vi "zero.out.and.convert.vi"(11 "Data":T1={"enabled"=[FALSE, FALSE, FALSE, FALSE, FALSE, FALSE, FALSE, FALSE], "byte"=[0, 0, 0, 0, 0, 0, 0, 0]} {"byte" format="%.0x"}) -> (2 "u64.be":u64 format="%.0x", 3 "Num.of.True":u8)   [LabVIEW 2020, in "fpganow.common.fpga.lvlib"]
uses:
  fpganow.common.fpga.lvlib
  u64.data.ctl
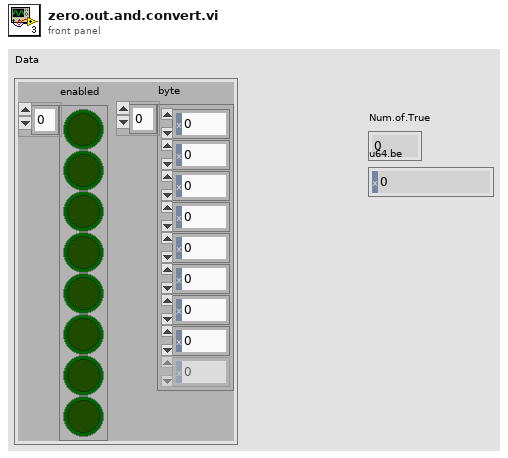
[diagram p1: front panel]
types:
  T1 = typedef "fpganow.common.fpga.lvlib/u64.data.ctl" = cluster{"enabled":bool[], "byte":u8[]}
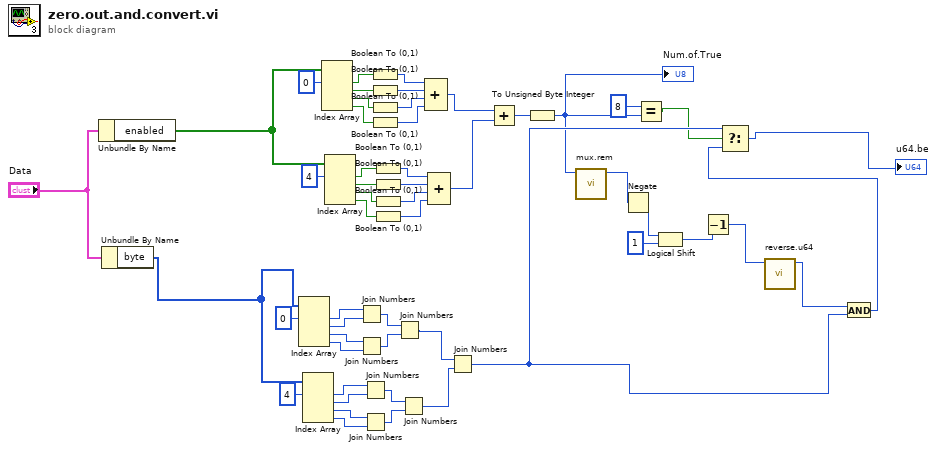
[diagram p0: block diagram]
diagram:
  n1 = Unbundle By Name("Data") -> ("enabled"=w31:bool[])
  n2 = Unbundle By Name("Data") -> ("byte"=w14:u8[])
  n3 = Index Array(array=w14, index #1=0 ("index")) -> (element #1=w29:u8, element #2=w28:u8, element #3=w27:u8, element #4=w26:u8)  [unwired: 3 in]
  n4 = Index Array(array=w14, index #1=4 ("index")) -> (element #1=w21:u8, element #2=w20:u8, element #3=w19:u8, element #4=w18:u8)  [unwired: 3 in]
  n5 = Index Array(array=w31, index #1=0 ("index")) -> (element #1=w33:bool, element #2=w35:bool, element #3=w37:bool, element #4=w40:bool)  [unwired: 3 in]
  n6 = Index Array(array=w31, index #1=4 ("index")) -> (element #1=w43:bool, element #2=w45:bool, element #3=w47:bool, element #4=w50:bool)  [unwired: 3 in]
  n7 = Join Numbers(hi=w29, lo=w28) -> ((hi.lo)=w25:u16)
  n8 = Join Numbers(hi=w27, lo=w26) -> ((hi.lo)=w24:u16)
  n9 = Join Numbers(hi=w21, lo=w20) -> ((hi.lo)=w17:u16)
  n10 = Join Numbers(hi=w19, lo=w18) -> ((hi.lo)=w16:u16)
  n11 = Boolean To (0,1)(Boolean=w33) -> (0, 1=w34:i16)
  n12 = Boolean To (0,1)(Boolean=w35) -> (0, 1=w36:i16)
  n13 = Boolean To (0,1)(Boolean=w37) -> (0, 1=w38:i16)
  n14 = Boolean To (0,1)(Boolean=w40) -> (0, 1=w39:i16)
  n15 = Boolean To (0,1)(Boolean=w43) -> (0, 1=w44:i16)
  n16 = Boolean To (0,1)(Boolean=w45) -> (0, 1=w46:i16)
  n17 = Boolean To (0,1)(Boolean=w47) -> (0, 1=w48:i16)
  n18 = Boolean To (0,1)(Boolean=w50) -> (0, 1=w49:i16)
  n19 = Join Numbers(hi=w25, lo=w24) -> ((hi.lo)=w23:u32)
  n20 = Join Numbers(hi=w17, lo=w16) -> ((hi.lo)=w15:u32)
  n21 = Compound Arithmetic op=ADD(w34, w36, w38, w39) -> (w41:i16)
  n22 = Compound Arithmetic op=ADD(w44, w46, w48, w49) -> (w51:i16)
  n23 = Join Numbers(hi=w23, lo=w15) -> ((hi.lo)=w5:u64)
  n24 = Add(x=w41, y=w51) -> (x+y=w52:i16)
  n25 = To Unsigned Byte Integer(number=w52) -> (unsigned 8bit integer=w4:u8)
  "Num.of.True" <- w4
  n26 = call "mux.rem.vi"("# of existing\nitems 3"=w4) -> ("y"=w11:i8)  [unwired: 10 in]
  n27 = Negate(x=w11) -> (-x=w10:i8)
  n28 = Equal?(x=u8 8, y=w4) -> (x = y?=w3:bool)
  n29 = Logical Shift(y=w10, x=u64 1) -> (x << y=w13:u64)
  n30 = Decrement(x=w13) -> (x-1=w9:u64)
  n31 = call "reverse.u64.vi"("U64.in"=w9) -> ("U64.reversed"=w8:u64)  [unwired: 10 in]
  n32 = And(x=w8, y=w5) -> (x .and. y?=w6:u64)
  n33 = Select(t=w5, s=w3, f=w6) -> (s? t:f=→"u64.be":u64)
